vi "ReadAppInputDataRequest.vi"(8 "error in (no error)":errorcluster, 10 "InputData":variant, 11 "ModuleID":i32=-1) -> (0 "error out":errorcluster)   [LabVIEW 2017, in "AppModule.lvlib"]
uses:
  AppModule.lvlib
  clEventType.ctl
  <vilib>/Utility/error.llb/Error Cluster From Error Code.vi
  <vilib>/ErrorRing/Error Ring.xnode
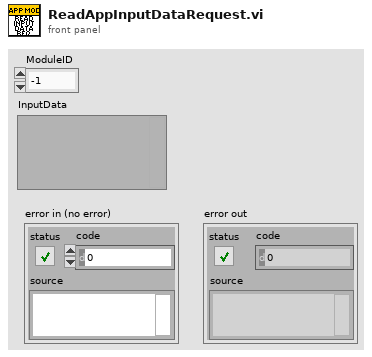
[diagram p1: front panel]
types:
  T1 = typedef "AppModule.lvlib/clRequestEvents.ctl" = cluster{"StopRequest":refnum<user-event>, "PathToINI":refnum<user-event>, " LoadPlugin":refnum<user-event>, "OpenAppConfig":refnum<user-event>, "WriteInputData":refnum<user-event>, "ReadInputData":refnum<user-event>, "GetAppOutput":refnum<user-event>, "WriteEvtConfig":refnum<user-event>, "WriteBcAppInfo":refnum<user-event>, "ReadBcAppInfo":refnum<user-event>, "AggregateRequest":refnum<user-event>, "WriteAppConfig":refnum<user-event>, "ReadAppConfig":refnum<user-event>, "CalcAppOutput":refnum<user-event>, "ShowPanel":refnum<user-event>}
  T2 = typedef "AppModule.lvlib/clEventType.ctl" = cluster{"ModuleID":i32, "Data":variant}
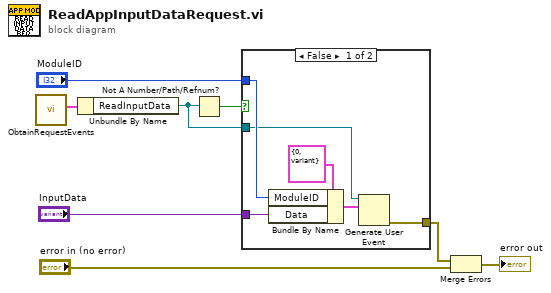
[diagram p0: block diagram]
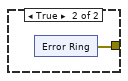
[diagram p2: hidden frame]
diagram:
  n1 = call "ObtainRequestEvents.vi"() -> ("clRequestEvents"=w8:T1)  [unwired: 10 in, 1 out]
  n2 = Unbundle By Name(w8) -> ("ReadInputData"=w5:refnum<user-event>)
  n3 = Not A Number/Path/Refnum?(number/path/refnum=w5) -> (NaN/Path/Refnum?=w7:bool)
  n4 = case shown="False" w7 {
    tunnel: "ModuleID" -> [w13 _]
    tunnel: w5 -> [w10 _]
    tunnel: "InputData" -> [w12 _]
    tunnel: [w9 w15] -> w2
    frame False {
      n5 = Bundle By Name(cluster=T2 {"ModuleID"=0, "Data"=variant} ("clEventType"), "ModuleID"=w13, "Data"=w12) -> (w11:T2)
      n6 = Generate User Event(user event=w10, event data cluster=w11) -> (error out=w9:errorcluster)  [unwired: 2 in, 1 out]
    }
    frame True {
      n7 = xnode "Error Ring"() -> ("error out"=w15:errorcluster)
    }
  }
  n8 = Merge Errors(w2, "error in (no error)") -> (→"error out":errorcluster)
